vi "Append Section Break to Report.vi"(0 "report in":refnum<class "NI_report.lvclass">, 11 "error in (no error)":errorcluster) -> (4 "report out":refnum<class "NI_report.lvclass">, 15 "error out":errorcluster)   [LabVIEW 2017, in "NI_report.lvclass"]
uses:
  <vilib>/Utility/NIReport.llb/NI_report.lvclass
  <vilib>/Utility/NIReport.llb/NI_ReportGenerationCore.lvlib
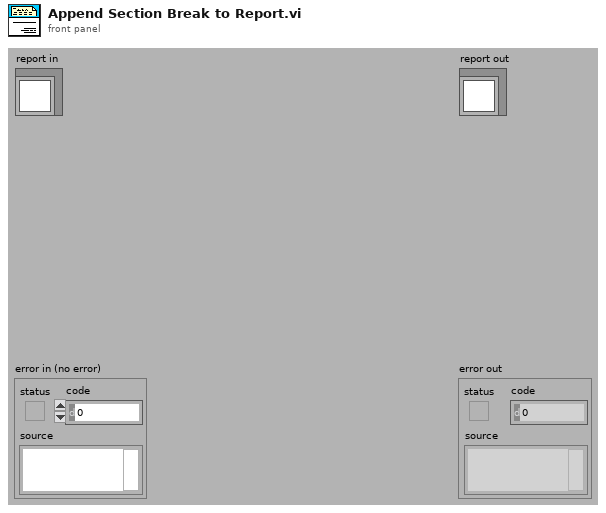
[diagram p1: front panel]
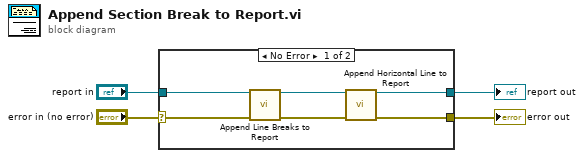
[diagram p0: block diagram]
diagram:
  n1 = case shown="No Error" "error in (no error)" {
    selector: "error in (no error)" -> [w6 w12]
    tunnel: [w5 w12] -> w3
    tunnel: [w9 w11] -> w1
    tunnel: "report in" -> [w10 w11]
    frame No Error {
      n2 = call <vilib>:"Append Line Breaks to Report.vi"("report in"=w10, "error in (no error)"=w6) -> ("report out"=w8:refnum<class "NI_report.lvclass">, "error out"=w7:errorcluster)  [unwired: 1 in, 11 out]
      n3 = call-dynamic "Append Horizontal Line to Report.vi"("report in"=w8, "error in (no error)"=w7) -> ("report out"=w9:refnum<class "NI_report.lvclass">, "error out"=w5:errorcluster)  [unwired: 6 in, 6 out]
    }
    frame Error {
    }
  }
  "error out" <- w3
  "report out" <- w1
